vi "ActionVIOnLoad.vi"(8 "error in (no error)":errorcluster, 11 "Device Item Ref in":T1 format="%.0x") -> (0 "error out":errorcluster, 3 "Device Item Ref out":T1 format="%.0x")   [LabVIEW 2019, in "Fuel Injector Analysis Addon System Explorer.lvlib"]
uses:
  Fuel Injector Analysis Addon System Explorer.lvlib
  <vilib>/NI VeriStand/Custom Device API/Custom Device Item Ref.ctl
  NationalInstruments.VeriStand.SystemDefinitionAPI
  Addon Shared/SubVIs/Constants.vi
  <vilib>/NI VeriStand/Custom Device Tools/Custom Device Utility Library/NI VeriStand - Search for Item by GUID.vi
  <vilib>/NI VeriStand/Custom Device Tools/Custom Device Utility Library/NI VeriStand - Search for All Items by GUID.vi
  <vilib>/NI VeriStand/Custom Device API/Set Item Property (Variant).vi
  <vilib>/NI VeriStand/Custom Device API/Custom Device API.lvlib
  <vilib>/NI VeriStand/Custom Device Tools/Custom Device Utility Library/Custom Device Utility Library.lvlib
  Addon Shared/Fuel Injector Analysis Addon Shared.lvlib
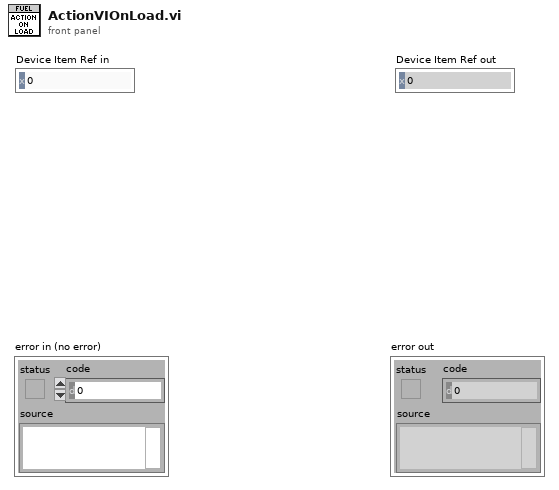
[diagram p1: front panel]
types:
  T1 = typedef "Custom Device API.lvlib/Custom Device Item Ref.ctl" = u64
  T2 = typedef "Fuel Injector Analysis Addon Shared.lvlib/Analysis.Channels.Select.ctl" = cluster{"Pull In Time":bool, "Pull In Max Current":bool, "Pull In Max Voltage":bool, "Pull In Min Voltage":bool, "Pull In Avg Voltage":bool, "Hold Time":bool, "Hold Max Current":bool, "Hold Min Current":bool, "Hold Avg Current":bool, "Hold Max Voltage":bool, "Hold Min Voltage":bool, "Hold Avg Max Voltage":bool, "Hold Avg Min Voltage":bool, "Off Time":bool, "Off Max Current":bool, "Off Min Current":bool, "Off Avg Current":bool, "Off Max Voltage":bool, "Off Min Voltage":bool, "Off Avg Voltage":bool, "Total Voltage Pulses":bool, "Total Stage Time":bool}
  T3 = typedef "Fuel Injector Analysis Addon Shared.lvlib/Register.Info.ctl" = cluster{"Name":string, "Data Type":T4, "Default Value":variant}
  T4 = typedef "Fuel Injector Analysis Addon Shared.lvlib/FPGA Data Types.ctl" = enum8{"<Null>", "Injector.Core.Setting", "Injector.Global.Setting", "Injector.Mux.Setting", "Injector.Timing"}
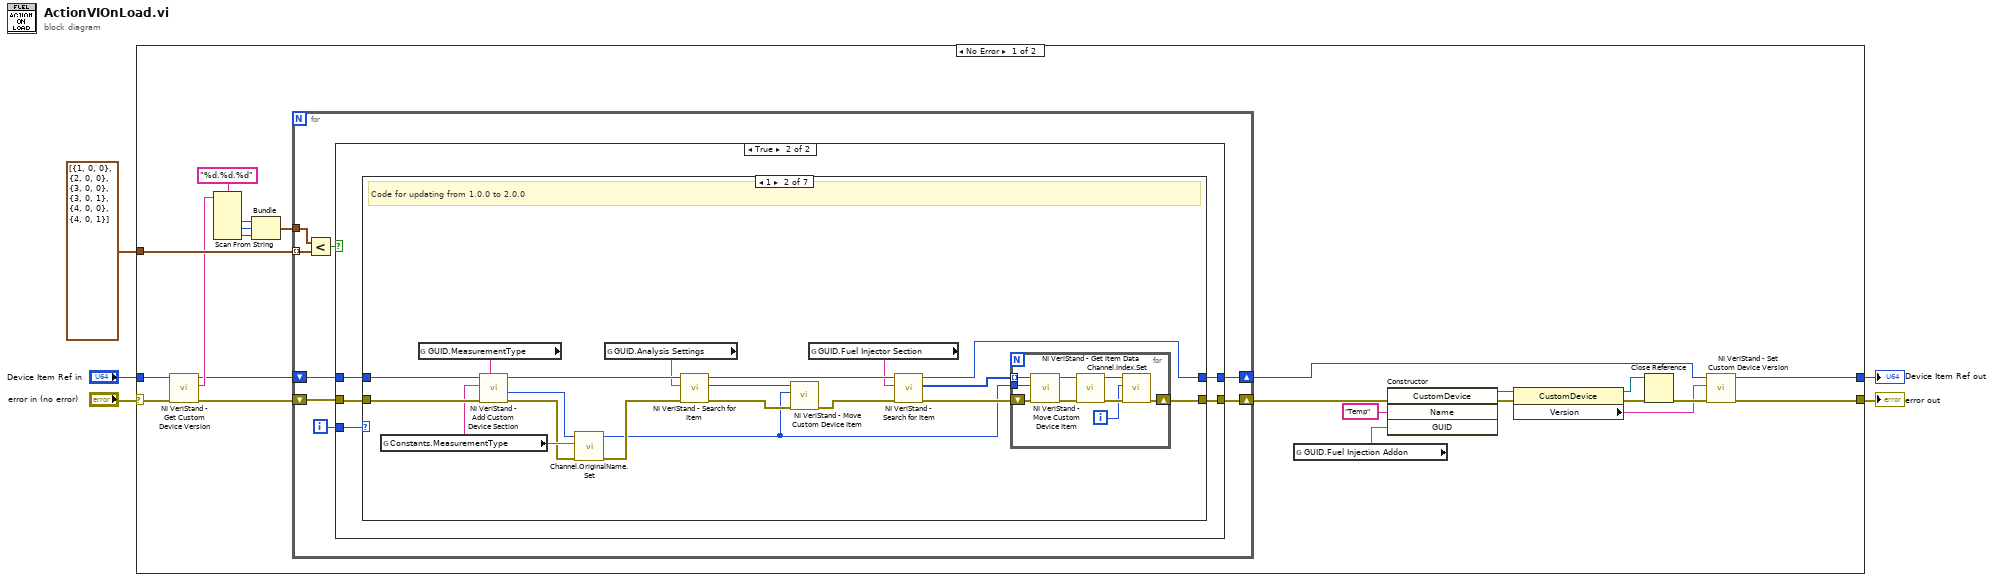
[diagram p0: block diagram]
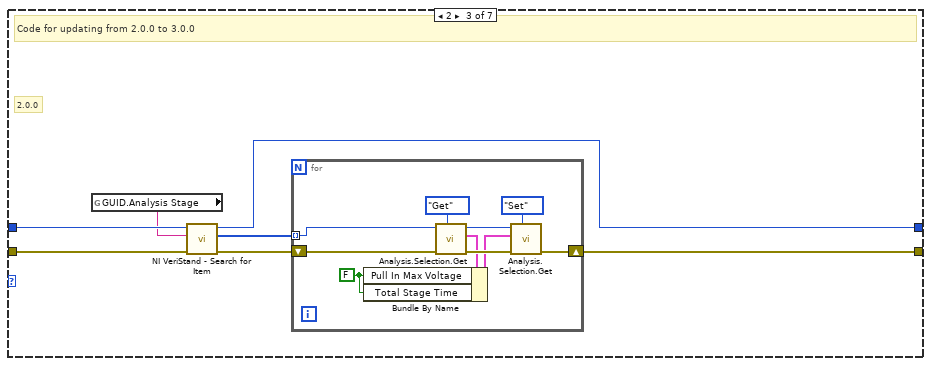
[diagram p4: hidden frame]
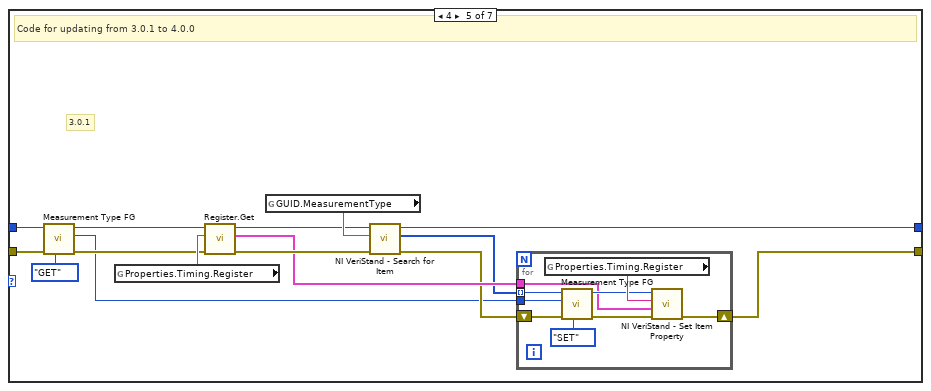
[diagram p6: hidden frame]
diagram:
  n1 = case shown="No Error" "error in (no error)" {
    selector: "error in (no error)" -> [w11 w122]
    tunnel: [w21 w122] -> w2
    tunnel: "Device Item Ref in" -> [w10 w121]
    tunnel: [w20 w121] -> w1
    tunnel: cluster{i32, i32, i32}[] [{1, 0, 0}, {2, 0, 0}, {3, 0, 0}, {3, 0, 1}, {4, 0, 0}, {4, 0, 1}] -> [w28 _]
    frame No Error {
      n2 = call <vilib>:"NI VeriStand - Get Custom Device Version.vi"("error in (no error)"=w11, "Device Ref in"=w10) -> ("error out"=w7:errorcluster, "Value"=w14:string, "Device Ref out"=w6:T1)  [unwired: 7 in]
      n3 = Scan From String(format string="%d.%d.%d", input string=w14) -> (output 1=w13:i32, output 2=w12:i32, output 3=w15:i32)  [unwired: 5 in, 3 out]
      n4 = Bundle(w13, w12, w15) -> (w8:cluster{i32, i32, i32})  [unwired: 1 in]
      n5 = for {
        tunnel: w28 -> [w32] mode=indexing
        shift-right: [w35] -> w19
        shift-left: w7 -> [w30]
        shift-right: [w34] -> w18
        shift-left: w6 -> [w29]
        tunnel: w8 -> [w31]
        i -> [w33]
        n6 = Less?(x=w31, y=w32) -> (x < y?=w36:bool)
        n7 = case shown="True" w36 {
          tunnel: w30 -> [w38 w43]
          tunnel: [w38 w42] -> w35
          tunnel: w29 -> [w37 w39]
          tunnel: [w37 w40] -> w34
          tunnel: w33 -> [_ w41]
          frame False {
          }
          frame True {
            n8 = case shown="1" w41 {
              tunnel: w43 -> [w45 w64 w80 w92 w97 w118 w120]
              tunnel: [w45 w58 w76 w92 w102 w118 w120] -> w42
              tunnel: [w44 w61 w74 w91 w101 w117 w119] -> w40
              tunnel: w39 -> [w44 w63 w79 w91 w95 w117 w119]
              frame 0 {
                # "Initial Onload"
              }
              frame 1 {
                # "Code for updating from 1.0.0 to 2.0.0"
                n9 = global read "Constants.vi" "Constants.MeasurementType"() -> (w50:string)
                n10 = global read "Constants.vi" "GUID.MeasurementType"() -> (w51:string)
                n11 = call <vilib>:"NI VeriStand - Add Custom Device Section.vi"("GUID (Default Section)"=w51, "error in (no error)"=w64, "Section Name"=w50, "Parent Ref in"=w63) -> ("error out"=w49:errorcluster, "Section Ptr"=w47:T1, "Parent Ref out"=w62:T1)  [unwired: 4 in, 1 out]
                n12 = call "Channel.OriginalName.Set.vi"("error in (no error)"=w49, "Constants.Channel Name"=w50, "Ref"=w47) -> ("error out"=w48:errorcluster, "Ref out"=w46:T1)  [unwired: 7 in]
                n13 = global read "Constants.vi" "GUID.Analysis Settings"() -> (w53:string)
                n14 = call-poly <vilib>:"NI VeriStand - Search for Item.vi"("error in"=w48, "Item GUID"=w53, "Section Ref in"=w62) -> ("error out"=w56:errorcluster, "Item Ref"=w57:T1, "Section Ref out"=w55:T1)  [unwired: 5 in, 1 out]
                n15 = call <vilib>:"NI VeriStand - Move Custom Device Item.vi"("error in (no error)"=w56, "New Parent Ref in"=w46, "Item Ref in"=w57) -> ("error out"=w54:errorcluster)  [unwired: 6 in, 2 out]
                n16 = global read "Constants.vi" "GUID.Fuel Injector Section"() -> (w52:string)
                n17 = call-poly <vilib>:"NI VeriStand - Search for Item.vi"("error in"=w54, "Item GUID"=w52, "Section Ref in"=w55) -> ("error out"=w59:errorcluster, "Item Refs"=w60:T1[], "Section Ref out"=w61:T1)  [unwired: 5 in, 1 out]
                n18 = for {
                  tunnel: w60 -> [w73] mode=indexing
                  shift-right: [w66] -> w58
                  shift-left: w59 -> [w72]
                  tunnel: w46 -> [w71]
                  i -> [w65]
                  n19 = call <vilib>:"NI VeriStand - Move Custom Device Item.vi"("error in (no error)"=w72, "New Parent Ref in"=w71, "Item Ref in"=w73) -> ("error out"=w69:errorcluster, "Item Ref out"=w70:T1)  [unwired: 6 in, 1 out]
                  n20 = call <vilib>:"NI VeriStand - Get Item Data.vi"("error in (no error)"=w69, "Item Ref in"=w70) -> ("error out"=w67:errorcluster, "Item Ref out"=w68:T1)  [unwired: 6 in, 2 out]
                  n21 = call "Channel.Index.Set.vi"("error in (no error)"=w67, "Constants.Index"=w65, "Ref"=w68) -> ("error out"=w66:errorcluster)  [unwired: 7 in, 1 out]
                }
              }
              frame 2 {
                # "2.0.0"
                # "Code for updating from 2.0.0 to 3.0.0"
                n22 = global read "Constants.vi" "GUID.Analysis Stage"() -> (w78:string)
                n23 = call-poly <vilib>:"NI VeriStand - Search for Item.vi"("error in"=w80, "Item GUID"=w78, "Section Ref in"=w79) -> ("error out"=w77:errorcluster, "Item Refs"=w75:T1[], "Section Ref out"=w74:T1)  [unwired: 5 in, 1 out]
                n24 = for {
                  shift-right: [w86] -> w76
                  shift-left: w77 -> [w88]
                  tunnel: w75 -> [w81] mode=indexing
                  w82 = FALSE ("Pull In Max Voltage")
                  n25 = call "Analysis.Selection.Get.vi"("Action"=enum8{"Get", "Set"}."Get", "error in (no error)"=w88, "Item Ref in"=w81) -> ("error out"=w87:errorcluster, "Selections"=w84:T2, "Item Ref out"=w85:T1)  [unwired: 6 in]
                  n26 = Bundle By Name(cluster=w84, "Pull In Max Voltage"=w82, "Total Stage Time"=w82) -> (w83:T2)
                  n27 = call "Analysis.Selection.Get.vi"("Action"=enum8{"Get", "Set"}."Set", "error in (no error)"=w87, "Selections"=w83, "Item Ref in"=w85) -> ("error out"=w86:errorcluster)  [unwired: 5 in, 2 out]
                }
              }
              frame 3 {
                # "3.0.0"
                # "Code for updating from 3.0.0 to 3.0.1"
              }
              frame 4 {
                # "3.0.1"
                # "Code for updating from 3.0.1 to 4.0.0"
                n28 = call "Measurement Type FG.vi"("Action"=enum8{"GET", "SET"}."GET", "error in (no error)"=w97, "Item Ref"=w95) -> ("error out"=w96:errorcluster, "Sample rate (S/s)"=w93:u32, "Item Ref out"=w94:T1)  [unwired: 6 in]
                n29 = global read "Constants.vi" "Properties.Timing.Register"() -> (w106:string)
                n30 = call "Register.Get.vi"("error in (no error)"=w96, "Property"=w106, "Section Ref in"=w94) -> ("error out"=w104:errorcluster, "Register"=w103:T3, "Item Ref out"=w105:T1)  [unwired: 6 in]
                n31 = global read "Constants.vi" "GUID.MeasurementType"() -> (w107:string)
                n32 = call-poly <vilib>:"NI VeriStand - Search for Item.vi"("error in"=w104, "Item GUID"=w107, "Section Ref in"=w105) -> ("error out"=w100:errorcluster, "Item Refs"=w99:T1[], "Section Ref out"=w101:T1)  [unwired: 5 in, 1 out]
                n33 = for {
                  tunnel: w103 -> [w112]
                  shift-right: [w111] -> w102
                  shift-left: w100 -> [w110]
                  tunnel: w99 -> [w109] mode=indexing
                  tunnel: w93 -> [w108]
                  n34 = global read "Constants.vi" "Properties.Timing.Register"() -> (w115:string)
                  n35 = call "Measurement Type FG.vi"("Action"=enum8{"GET", "SET"}."SET", "error in (no error)"=w110, "Sample rate (S/s)"=w108, "Item Ref"=w109) -> ("error out"=w114:errorcluster, "Item Ref out"=w113:T1)  [unwired: 5 in, 1 out]
                  n36 = call-poly <vilib>:"NI VeriStand - Set Item Property.vi"("error in (no error)"=w114, "Value"=w112, "Property Name"=w115, "Item Ref in"=w113) -> ("error out"=w111:errorcluster)  [unwired: 5 in, 2 out]
                }
              }
              frame 5 {
                # "4.0.0"
                # "Code for updating from 4.0.0 to 4.0.1"
              }
              frame Default {
                # "Nothing to update"
              }
            }
          }
        }
      }
      n37 = global read "Constants.vi" "GUID.Fuel Injection Addon"() -> (w16:string)
      n38 = constructor class="CustomDevice"(error in=w19, "Name"="Temp", "GUID"=w16) -> (reference out=w27:refnum<k24>, error out=w26:errorcluster)  [unwired: 2 in, 3 out]
      n39 = property class="CustomDevice"(reference=w27, error in=w26) -> (reference out=w24:refnum<k24>, error out=w25:errorcluster, "Version"=w22:string)
      n40 = Close Reference(reference=w24, error in (no error)=w25) -> (error out=w23:errorcluster)
      n41 = call <vilib>:"NI VeriStand - Set Custom Device Version.vi"("error in (no error)"=w23, "Value"=w22, "Device Ref in"=w18) -> ("error out"=w21:errorcluster, "Device Ref out"=w20:T1)  [unwired: 7 in]
    }
    frame Error {
    }
  }
  "error out" <- w2
  "Device Item Ref out" <- w1
